vi "heuristic.vi"(10 "pos":i32[][](array[numeric]), 11 "exist":i32[][](array[numeric])) -> (3 "heuristic":dbl)   [LabVIEW 2022 SP3, in "subvis.lvlib"]
uses:
  subvis.lvlib
panel:
  out "availableBlue":i32[][](array[numeric])
  out "availableRed":i32[][](array[numeric])
  out "blueMoves":i32
  out "redMoves":i32
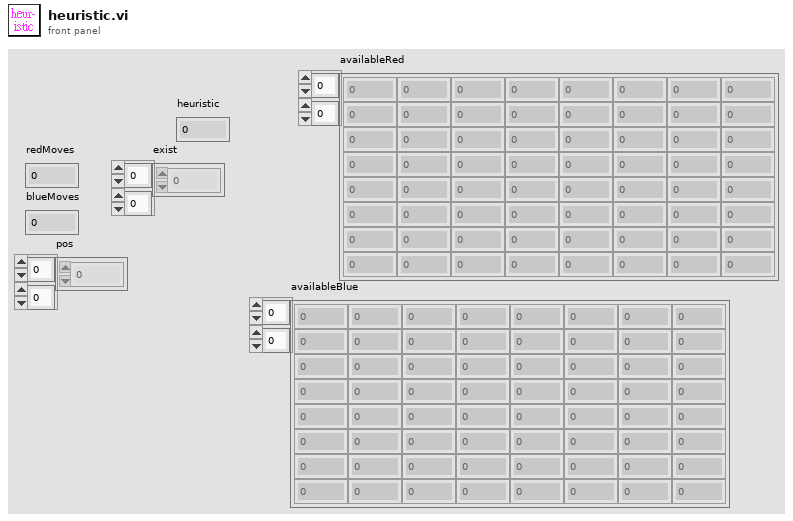
[diagram p1: front panel]
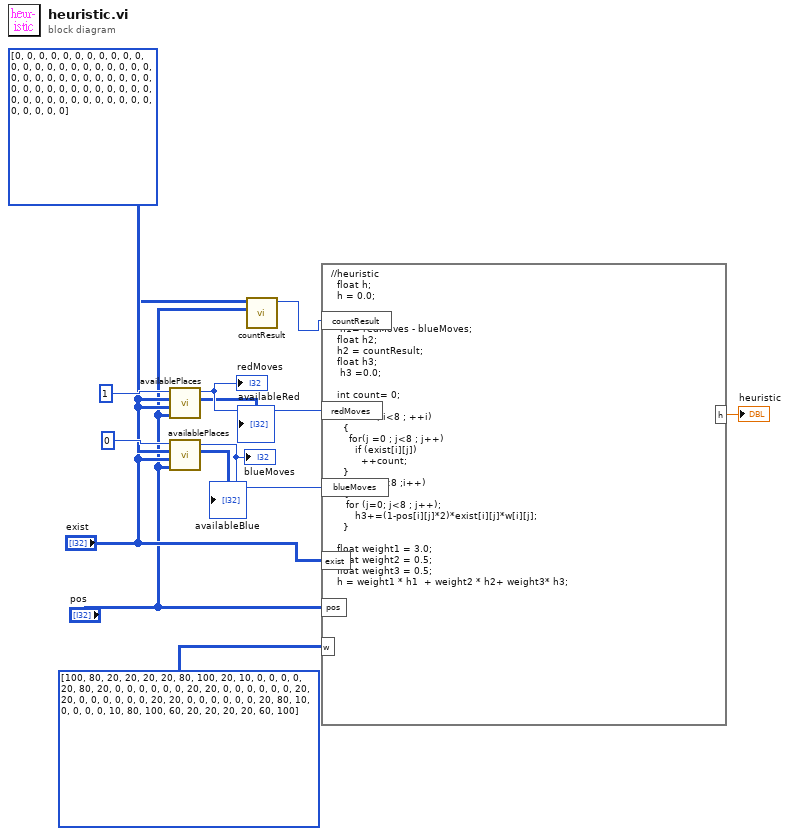
[diagram p0: block diagram]
diagram:
  w6 = i32[][] [[0, 0, 0, 0, 0, 0, 0, 0], [0, 0, 0, 0, 0, 0, 0, 0], [0, 0, 0, 0, 0, 0, 0, 0], [0, 0, 0, 0, 0, 0, 0, 0], [0, 0, 0, 0, 0, 0, 0, 0], [0, 0, 0, 0, 0, 0, 0, 0], [0, 0, 0, 0, 0, 0, 0, 0], [0, 0, 0, 0, 0, 0, 0, 0]] ("w")
  n1 = call "availablePlaces.vi"("pos"="pos", "exist"="exist", "available"=w6, "redTurn"=u8 1) -> ("availableNew"=→"availableRed":i32[][], "count"=w10:i32)  [unwired: 4 in, 2 out]
  "redMoves" <- w10
  n2 = call "availablePlaces.vi"("pos"="pos", "exist"="exist", "available"=w6, "redTurn"=u8 0) -> ("availableNew"=→"availableBlue":i32[][], "count"=w9:i32)  [unwired: 4 in, 2 out]
  "blueMoves" <- w9
  n3 = call "countResult.vi"("pos"="pos", "exist"="exist") -> ("result"=w5:i32)  [unwired: 9 in]
  n4 = formula code="//heuristic\n  float h; \n  h = 0.0;\n\n  float h1; \n   h1= redMoves - blueMoves;\n  float h2;\n  h2 = countResult;\n  float h3;\n   h3 =0.0;\n  \n  int count= 0;\nint i;int j;\n  for (i =0; i<8 ; ++i)\n    {\n      for(j =0 ; j<8 ; j++)\n        if (exist[i][j])\n          ++count;\n    }\n  for (i=0; i<8 ;i++)\n    {\n     for (j=0; j<8 ; j++);\n        h3+=(1-pos[i][j]*2)*exist[i][j]*w[i][j];\n    }\n\n  float weight1 = 3.0;\n  float weight2 = 0.5; \n  float weight3 = 0.5; \n  h = weight1 * h1  + weight2 * h2+ weight3* h3;"("redMoves"=w10, "blueMoves"=w9, "exist"="exist", "pos"="pos", "countResult"=w5, "w"=i32[][] [[100, 80, 20, 20, 20, 20, 80, 100], [20, 10, 0, 0, 0, 0, 20, 80], [20, 0, 0, 0, 0, 0, 0, 20], [20, 0, 0, 0, 0, 0, 0, 20], [20, 0, 0, 0, 0, 0, 0, 20], [20, 0, 0, 0, 0, 0, 0, 20], [80, 10, 0, 0, 0, 0, 10, 80], [100, 60, 20, 20, 20, 20, 60, 100]]) -> ("h"=→"heuristic":dbl)
